vi "Set Queues.vi"(10 "Queues":T1, 11 "Queues in":refnum<class "Queues.lvclass">) -> (3 "Queues out":refnum<class "Queues.lvclass">)   [LabVIEW 2021, in "jettl.lvlib" / "jettl Queue Actor.lvlib" / "Queues.lvclass"]
uses:
  Queues.lvclass
  Queues.ctl
  Actor/Msg/Msg.lvclass
  Queues.lvclass/Queues.ctl
  jettl Queue Actor.lvlib
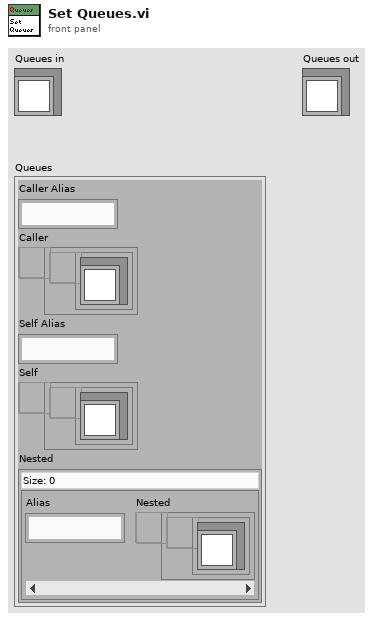
[diagram p1: front panel]
types:
  T1 = typedef "jettl.lvlib/jettl Queue Actor.lvlib/Queues.ctl" = cluster{"Caller Alias":string, "Caller":refnum<data-value>, "Self Alias":string, "Self":refnum<data-value>, "Nested":map{string, refnum<data-value>}}
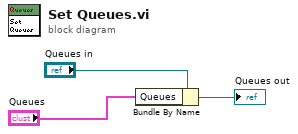
[diagram p0: block diagram]
diagram:
  n1 = Bundle By Name(cluster="Queues in", "Queues"="Queues") -> (→"Queues out":refnum<class "Queues.lvclass">)
